vi "Set Init Menu.vi"(8 "error in (no error)":errorcluster, 11 "Menu in":refnum<k9>) -> (3 "Menu out":refnum<k9>)   [LabVIEW 2016, in "CML UI.lvlib"]
uses:
  CML UI.lvlib
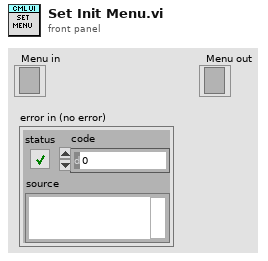
[diagram p1: front panel]
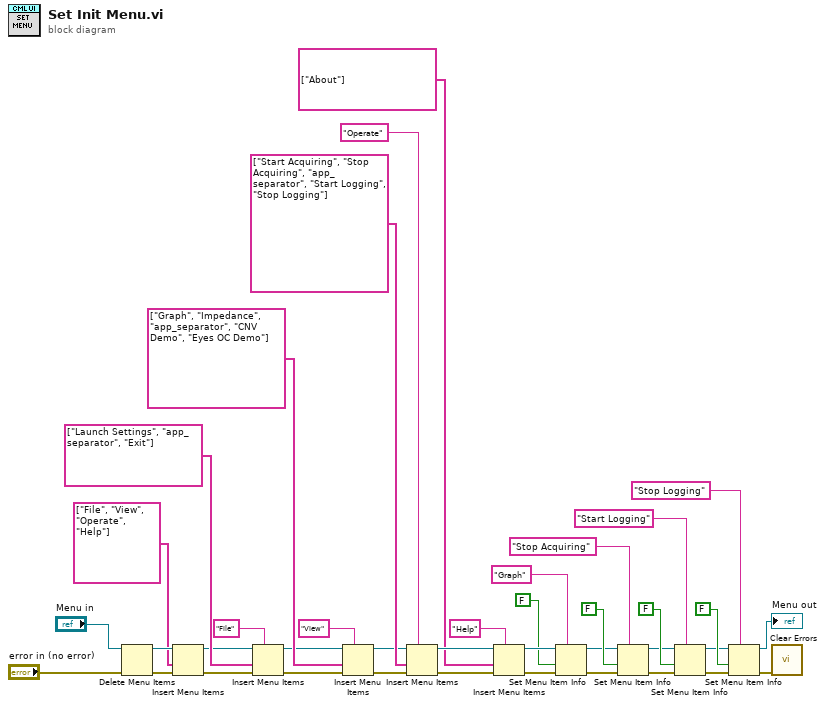
[diagram p0: block diagram]
diagram:
  n1 = Delete Menu Items(6:"error in (no error)", 9:"Menu in") -> (0:w28:errorcluster, 3:w25:refnum<k9>)  [unwired: 2 in]
  n2 = Insert Menu Items(6:w28, 7:string[] ["File", "View", "Operate", "Help"] ("L10n_item tags 1"), 9:w25) -> (0:w27:errorcluster, 3:w23:refnum<k9>)  [unwired: 3 in, 1 out]
  n3 = Insert Menu Items(5:"File" ("L10n_menu tag"), 6:w27, 7:string[] ["Launch Settings", "app_separator", "Exit"] ("L10n_item tags 2"), 9:w23) -> (0:w34:errorcluster, 3:w33:refnum<k9>)  [unwired: 2 in, 1 out]
  n4 = Insert Menu Items(5:"View" ("L10n_menu tag"), 6:w34, 7:string[] ["Graph", "Impedance", "app_separator", "CNV Demo", "Eyes OC Demo"] ("L10n_item tags 2"), 9:w33) -> (0:w38:errorcluster, 3:w37:refnum<k9>)  [unwired: 2 in, 1 out]
  n5 = Insert Menu Items(5:"Operate" ("L10n_menu tag"), 6:w38, 7:string[] ["Start Acquiring", "Stop Acquiring", "app_separator", "Start Logging", "Stop Logging"] ("L10n_item tags 2"), 9:w37) -> (0:w20:errorcluster, 3:w21:refnum<k9>)  [unwired: 2 in, 1 out]
  n6 = Insert Menu Items(5:"Help" ("L10n_menu tag"), 6:w20, 7:string[] ["About"] ("L10n_item tags 2"), 9:w21) -> (0:w16:errorcluster, 3:w18:refnum<k9>)  [unwired: 2 in, 1 out]
  n7 = Set Menu Item Info(7:"Graph" ("item tag"), 8:w16, 9:FALSE ("enabled"), 11:w18) -> (0:w11:errorcluster, 3:w12:refnum<k9>)  [unwired: 3 in]
  n8 = Set Menu Item Info(7:"Stop Acquiring" ("item tag"), 8:w11, 9:FALSE ("enabled"), 11:w12) -> (0:w7:errorcluster, 3:w8:refnum<k9>)  [unwired: 3 in]
  n9 = Set Menu Item Info(7:"Start Logging" ("item tag"), 8:w7, 9:FALSE ("enabled"), 11:w8) -> (0:w3:errorcluster, 3:w4:refnum<k9>)  [unwired: 3 in]
  n10 = Set Menu Item Info(7:"Stop Logging" ("item tag"), 8:w3, 9:FALSE ("enabled"), 11:w4) -> (0:w1:errorcluster, 3:→"Menu out":refnum<k9>)  [unwired: 3 in]
  n11 = call <vilib>:"Clear Errors.vi"("error in (no error)"=w1) -> ()  [unwired: 5 in, 2 out]
